vi "GUI Alarms Tbl.vi"(0 "data in":T1={"alarms"=[{"obj_tag"="AI0", "event_tag"="AI0.OUT_OF_RANGE_MIN", "Description"="Уровень  масла (НС очистки и охлаждения). Вне диапазона (низкий уровень)", "ALARM TYPE"=enum."Alarm", "Value DBL"=0.0, "Value INT"=1, "Value STR"="Alarm", "Time Stamp"=timestamp(3830845009.237916 s since 1904-01-01)}, {"obj_tag"="AI1", "event_tag"="AI1.OUT_OF_RANGE_MIN", "Description"="Уровень масла (НС подачи масла). Вне диапазона (низкий уровень)", "ALARM TYPE"=enum."Alarm", "Value DBL"=0.0, "Value INT"=1, "Value STR"="Alarm", "Time Stamp"=timestamp(3830845009.237916 s since 1904-01-01)}, {"obj_tag"="AI10", "event_tag"="AI10.OUT_OF_RANGE_MIN", "Description"="Датчик давления в линии измерения утечек. Вне диапазона (низкий уровень)", "ALARM TYPE"=enum."Alarm", "Value DBL"=0.0, "Value INT"=1, "Value STR"="Alarm", "Time Stamp"=timestamp(3830845009.237916 s since 1904-01-01)}, {"obj_tag"="AI2", "event_tag"="AI2.OUT_OF_RANGE_MIN", "Description"="Температура масла (НС очистки и охлаждения). Вне диапазона (низкий уровень)", "ALARM TYPE"=enum."Alarm", "Value DBL"=0.0, "Value INT"=1, "Value STR"="Alarm", "Time Stamp"=timestamp(3830845009.237916 s since 1904-01-01)}, {"obj_tag"="AI3", "event_tag"="AI3.OUT_OF_RANGE_MIN", "Description"="Температура масла (НС подачи масла). Вне диапазона (низкий уровень)", "ALARM TYPE"=enum."Alarm", "Value DBL"=0.0, "Value INT"=1, "Value STR"="Alarm", "Time Stamp"=timestamp(3830845009.237916 s since 1904-01-01)}, {"obj_tag"="AI4", "event_tag"="AI4.OUT_OF_RANGE_MIN", "Description"="Обратная связь от клапана регулировки низкого давления . Вне диапазона (низкий уровень)", "ALARM TYPE"=enum."Alarm", "Value DBL"=0.0, "Value INT"=1, "Value STR"="Alarm", "Time Stamp"=timestamp(3830845009.237916 s since 1904-01-01)}, {"obj_tag"="AI5", "event_tag"="AI5.OUT_OF_RANGE_MIN", "Description"="Давление после насоса ВД. Вне диапазона (низкий уровень)", "ALARM TYPE"=enum."Alarm", "Value DBL"=0.0, "Value INT"=1, "Value STR"="Alarm", "Time Stamp"=timestamp(3830845009.237916 s since 1904-01-01)}, {"obj_tag"="AI6", "event_tag"="AI6.OUT_OF_RANGE_MIN", "Description"="Давление в образце. Вне диапазона (низкий уровень)", "ALARM TYPE"=enum."Alarm", "Value DBL"=0.0, "Value INT"=1, "Value STR"="Alarm", "Time Stamp"=timestamp(3830845009.237916 s since 1904-01-01)}, {"obj_tag"="AI7", "event_tag"="AI7.OUT_OF_RANGE_MIN", "Description"="Давление в камере. Вне диапазона (низкий уровень)", "ALARM TYPE"=enum."Alarm", "Value DBL"=0.0, "Value INT"=1, "Value STR"="Alarm", "Time Stamp"=timestamp(3830845009.237916 s since 1904-01-01)}, {"obj_tag"="AI8", "event_tag"="AI8.OUT_OF_RANGE_MIN", "Description"="Давление  в  линии подачи воздуха в  БПВ. Вне диапазона (низкий уровень)", "ALARM TYPE"=enum."Alarm", "Value DBL"=0.0, "Value INT"=1, "Value STR"="Alarm", "Time Stamp"=timestamp(3830845009.237916 s since 1904-01-01)}, {"obj_tag"="AI9", "event_tag"="AI9.OUT_OF_RANGE_MIN", "Description"="Давление  в  линии подачи воздуха после БПВ. Вне диапазона (низкий уровень)", "ALARM TYPE"=enum."Alarm", "Value DBL"=0.0, "Value INT"=1, "Value STR"="Alarm", "Time Stamp"=timestamp(3830845009.237916 s since 1904-01-01)}, {"obj_tag"="M12", "event_tag"="M12.AUTOMAT_ERROR", "Description"="Двигатель перекачки. Выключен автомат", "ALARM TYPE"=enum."Alarm", "Value DBL"=1.0, "Value INT"=1, "Value STR"="Alarm", "Time Stamp"=timestamp(3830845009.739716 s since 1904-01-01)}, {"obj_tag"="M21", "event_tag"="M21.AUTOMAT_ERROR", "Description"="Двигатель подачи масла. Выключен автомат", "ALARM TYPE"=enum."Alarm", "Value DBL"=1.0, "Value INT"=1, "Value STR"="Alarm", "Time Stamp"=timestamp(3830845009.739716 s since 1904-01-01)}, {"obj_tag"="M22", "event_tag"="M22.AUTOMAT_ERROR", "Description"="Двигатель охлаждения. Выключен автомат", "ALARM TYPE"=enum."Alarm", "Value DBL"=1.0, "Value INT"=1, "Value STR"="Alarm", "Time Stamp"=timestamp(3830845009.739716 s since 1904-01-01)}]}, 1 "Multicolumn Listbox ref":refnum<vi>) -> (4 "alarms":bool, 6 "warning":bool)   [LabVIEW 2019]
uses:
  Logger_class/Current Alarms.ctl
  Logger_class/EventData.ctl
  TypeDef/AlarmType.ctl
  <vilib>/Utility/miscctls.llb/LVRowAndColumnTypeDef.ctl
  4dc6950c-d20f-47f8-a777-121e9da7eb0f.vi
panel:
  in  "error in":errorcluster
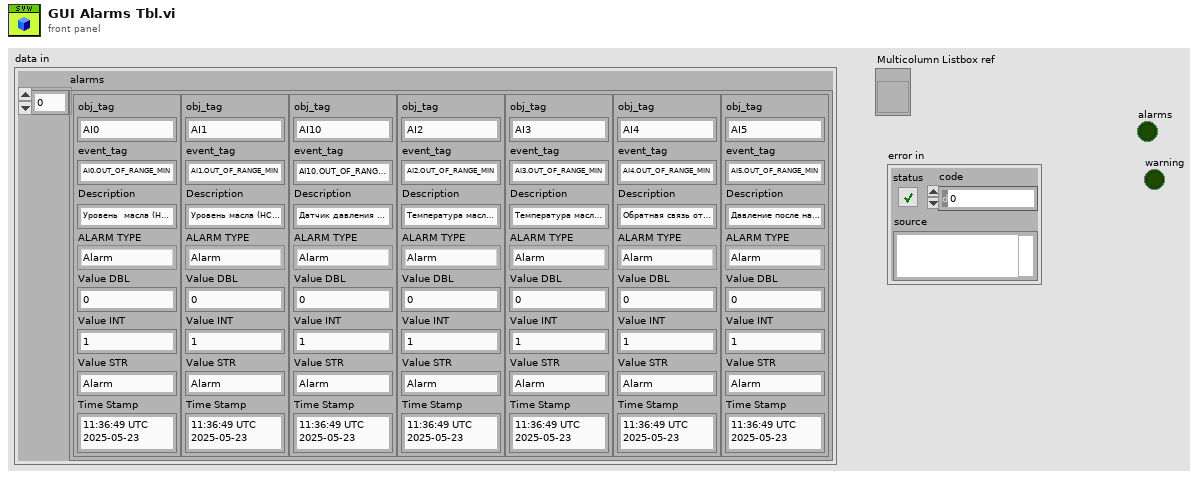
[diagram p1: front panel]
types:
  T1 = typedef "Current Alarms.ctl" = cluster{"alarms":T2[]}
  T2 = typedef "EventData.ctl" = cluster{"obj_tag":string, "event_tag":string, "Description":string, "ALARM TYPE":T3, "Value DBL":dbl, "Value INT":i32, "Value STR":string, "Time Stamp":timestamp}
  T3 = typedef "AlarmType.ctl" = enum16{"Normal", "Warning", "Alarm"}
  T4 = typedef "LVRowAndColumnTypeDef.ctl" = cluster{"Row":i32, "Column":i32}
  T5 = cluster{"ALARM TYPE":T3, "Time Stamp":timestamp, "Event":T2}
  T6 = cluster{"ALARM TYPE":T3, "Time Stamp":timestamp, "Event":T2}[]
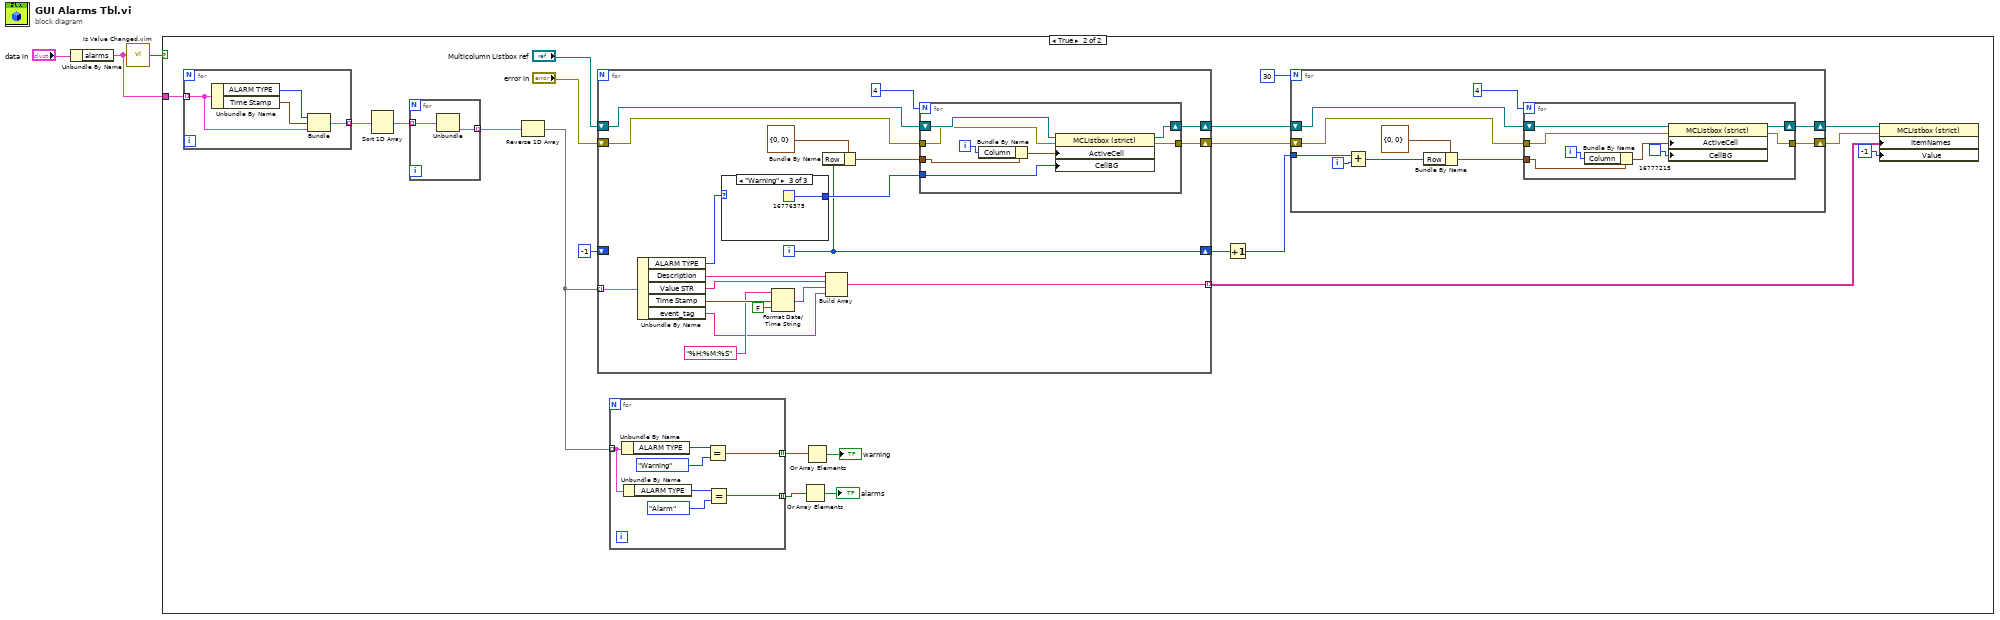
[diagram p0: block diagram]
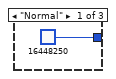
[diagram p3: hidden frame]
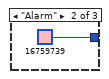
[diagram p4: hidden frame]
diagram:
  n1 = Unbundle By Name("data in") -> ("alarms"=w2:T2[])
  n2 = call "Is Value Changed.vim"("value"=w2) -> ("changed or first call?"=w1:bool)
  n3 = case shown="True" w1 {
    tunnel: w2 -> [_ w12]
    frame False {
    }
    frame True {
      n4 = for {
        tunnel: w12 -> [w55] mode=indexing
        tunnel: [w52] -> w22 mode=indexing
        n5 = Unbundle By Name(w55) -> ("ALARM TYPE"=w53:T3, "Time Stamp"=w54:timestamp)
        n6 = Bundle("ALARM TYPE"=w53, "Time Stamp"=w54, "Event"=w55) -> (w52:T5)  [unwired: 1 in]
      }
      n7 = Sort 1D Array(array=w22) -> (sorted array=w21:T6)
      n8 = for {
        tunnel: w21 -> [w51] mode=indexing
        tunnel: [w50] -> w20 mode=indexing
        n9 = Unbundle(w51) -> ("Event"=w50:T2)  [unwired: 2 out]
      }
      n10 = Reverse 1D Array(array=w20) -> (reversed array=w8:T2[])
      n11 = for {
        tunnel: w8 -> [w74] mode=indexing
        tunnel: [w70] -> w24 mode=indexing
        shift-right: [w66] -> w14
        shift-left: "Multicolumn Listbox ref" -> [w67]
        shift-right: [w65] -> w16
        shift-left: "error in" -> [w64]
        shift-right: [w56] -> w17
        shift-left: -1 -> [_]
        i -> [w56]
        n12 = Unbundle By Name(w74) -> ("ALARM TYPE"=w60:T3, "Description"=w72:string, "Value STR"=w58:string, "Time Stamp"=w73:timestamp, "event_tag"=w57:string)
        n13 = case shown="\"Warning\"" w60 {
          tunnel: [u32 16448250 u32 16759739 u32 16776375] -> w59
          frame "Normal" {
          }
          frame "Alarm" {
          }
          frame "Warning" {
          }
        }
        n14 = Format Date/Time String(time format string (%c)="%H:%M:%S", seconds (now)=w73, UTC format=FALSE) -> (date/time string=w71:string)
        n15 = Bundle By Name(cluster=T4 {"Row"=0, "Column"=0} ("Active Cell:Active Cell"), "Row"=w56) -> (w61:T4)
        n16 = Build Array(w72, w58, w71, w57) -> (w70:string[])
        n17 = for {
          N: 4 -> [_]
          tunnel: [w83] -> w65
          tunnel: w64 -> [w82]
          shift-right: [w84] -> w66
          shift-left: w67 -> [w85]
          tunnel: w61 -> [w81]
          tunnel: w59 -> [w78]
          i -> [w79]
          n18 = Bundle By Name(cluster=w81, "Column"=w79) -> (w80:T4)
          n19 = property class="MCListbox (strict)"(reference=w85, error in=w82, "ActiveCell"=w80, "CellBG"=w78) -> (reference out=w84:refnum<vi>, error out=w83:errorcluster)
        }
      }
      n20 = for {
        tunnel: w8 -> [w26] mode=indexing
        tunnel: [w29] -> w7 mode=indexing
        tunnel: [w25] -> w4 mode=indexing
        n21 = Unbundle By Name(w26) -> ("ALARM TYPE"=w31:T3)
        n22 = Unbundle By Name(w26) -> ("ALARM TYPE"=w27:T3)
        n23 = Equal?(x=w31, y=AlarmType."Warning") -> (x = y?=w29:bool)
        n24 = Equal?(x=w27, y=AlarmType."Alarm") -> (x = y?=w25:bool)
      }
      n25 = Or Array Elements(Boolean array=w4) -> (logical OR=→"alarms":bool)
      n26 = Or Array Elements(Boolean array=w7) -> (logical OR=→"warning":bool)
      n27 = Increment(x=w17) -> (x+1=w13:i32)
      n28 = for {
        N: 30 -> [_]
        shift-right: [w40] -> w10
        shift-left: w14 -> [w41]
        shift-right: [w39] -> w15
        shift-left: w16 -> [w38]
        tunnel: w13 -> [w32]
        i -> [w34]
        n29 = Add(x=w32, y=w34) -> (x+y=w33:i32)
        n30 = Bundle By Name(cluster=T4 {"Row"=0, "Column"=0} ("Active Cell:Active Cell"), "Row"=w33) -> (w35:T4)
        n31 = for {
          N: 4 -> [_]
          tunnel: [w47] -> w39
          tunnel: w38 -> [w46]
          shift-right: [w48] -> w40
          shift-left: w41 -> [w49]
          tunnel: w35 -> [w45]
          i -> [w43]
          n32 = Bundle By Name(cluster=w45, "Column"=w43) -> (w44:T4)
          n33 = property class="MCListbox (strict)"(reference=w49, error in=w46, "ActiveCell"=w44, "CellBG"=u32 16777215) -> (reference out=w48:refnum<vi>, error out=w47:errorcluster)
        }
      }
      n34 = property class="MCListbox (strict)"(reference=w10, error in=w15, "ItemNames"=w24, "Value"=-1) -> ()  [unwired: 2 out]
    }
  }
